vi "remove.issue.from.creator.map.vi"(10 "issue id":i32, 11 "creator map in":T1(c390)) -> (3 "creator map out":T1(c390))   [LabVIEW 2024, in "manager_daemon.lvclass"]
uses:
  manager_daemon.lvclass
  manager_daemon.lvclass/manager_daemon.ctl
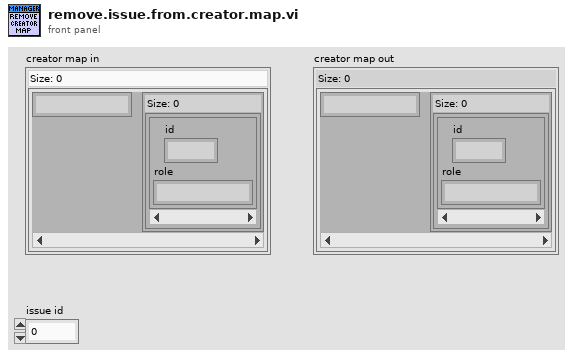
[diagram p1: front panel]
types:
  T1 = map{string, set{cluster{"id":i32, "role":string}}}
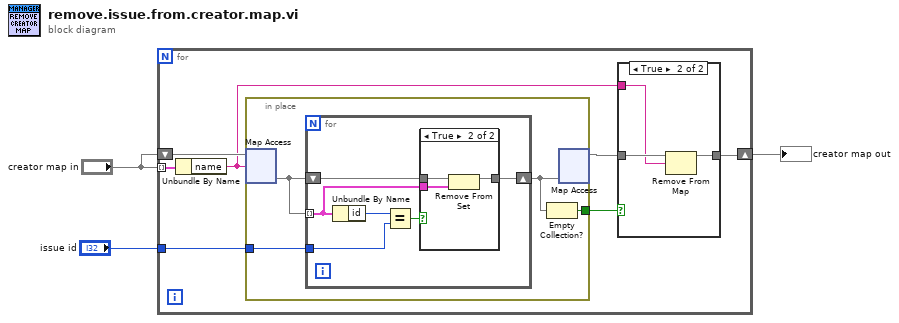
[diagram p0: block diagram]
diagram:
  n1 = for {
    tunnel: "creator map in" -> [w10] mode=indexing
    tunnel: "issue id" -> [w8]
    shift-right: [w6] -> w3
    shift-left: "creator map in" -> [w9]
    n2 = Unbundle By Name(w10) -> ("name"=w5:string)
    n3 = in-place {
      in-place-border: w8 -> [w17]
      in-place-border: [w15] -> w4
      n4 = in-place-map #1(w9, w5) -> (w18:set{cluster{"id":i32, "role":string}})  [unwired: 1 in, 1 out]
      n5 = for {
        tunnel: w18 -> [w19] mode=indexing
        shift-right: [w20] -> w16
        shift-left: w18 -> [w21]
        tunnel: w17 -> [w23]
        n6 = Unbundle By Name(w19) -> ("id"=w24:i32)
        n7 = Equal?(x=w24, y=w23) -> (x = y?=w22:bool)
        n8 = case shown="True" w22 {
          tunnel: w21 -> [w25 w28]
          tunnel: [w25 w27] -> w20
          tunnel: w19 -> [_ w26]
          frame False {
          }
          frame True {
            n9 = Remove From Set(10:w26, 11:w28) -> (3:w27:set{cluster{"id":i32, "role":string}})  [unwired: 1 out]
          }
        }
      }
      n10 = Empty Collection?(1:w16) -> (0:w15:bool)
      n11 = in-place-map #1(w16) -> (w7:T1)  [unwired: 1 in, 2 out]
    }
    n12 = case shown="True" w4 {
      tunnel: w7 -> [w11 w14]
      tunnel: [w11 w13] -> w6
      tunnel: w5 -> [_ w12]
      frame False {
      }
      frame True {
        n13 = Remove From Map(10:w12, 11:w14) -> (3:w13:T1)  [unwired: 2 out]
      }
    }
  }
  "creator map out" <- w3
